vi "Run OnNewStep.vi"(8 "error in (no error)":errorcluster, 11 "Step in":refnum<class "Step.lvclass">) -> (0 "error out":errorcluster, 2 "Change?":bool, 3 "Step out":refnum<class "Step.lvclass">)   [LabVIEW 2020, in "TSnax.lvlib" / "Step.lvclass"]
uses:
  Step.lvclass
  Step.lvclass/Step.ctl
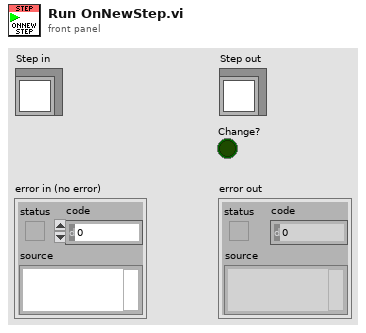
[diagram p1: front panel]
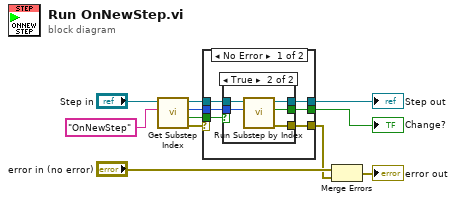
[diagram p0: block diagram]
diagram:
  n1 = call "Get Substep Index.vi"("Substep Name"="OnNewStep" ("arrayIndex"), "Step in"="Step in") -> ("error out"=w6:errorcluster, "Has Named Substep?"=w7:bool, "Index"=w5:i32, "Step out"=w4:refnum<class "Step.lvclass">)  [unwired: 6 in]
  n2 = case shown="No Error" w6 {
    selector: w6 -> [_ w24]
    tunnel: w7 -> [w17 _]
    tunnel: w5 -> [w16 _]
    tunnel: w4 -> [w15 w25]
    tunnel: [w14 w24] -> w1
    tunnel: [w13 _] -> w3
    tunnel: [w12 w25] -> w2
    frame No Error {
      n3 = case shown="True" w17 {
        tunnel: w16 -> [_ w22]
        tunnel: w15 -> [w18 w23]
        tunnel: [_ w21] -> w14
        tunnel: [_ w20] -> w13
        tunnel: [w18 w19] -> w12
        frame False {
        }
        frame True {
          n4 = call "Run Substep by Index.vi"("Substep Index"=w22, "Step in"=w23) -> ("error out"=w21:errorcluster, "Change?"=w20:bool, "Step out"=w19:refnum<class "Step.lvclass">)  [unwired: 7 in]
        }
      }
    }
    frame Error {
    }
  }
  "Step out" <- w2
  "Change?" <- w3
  n5 = Merge Errors("error in (no error)", w1) -> (→"error out":errorcluster)
